vi "Remove All Trailing Zeros.vi"(1 "String in":string) -> (0 "String out":string)   [LabVIEW 2020, in "eec EST 300.lvlib"]
doc: "This utility vi takes a list of ASCII floating point numbers and removes the trailing zeros from each number."
uses:
  <instrlib>/eec EST 300/eec EST 300.lvlib
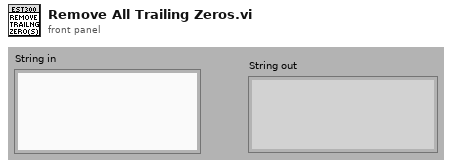
[diagram p1: front panel]
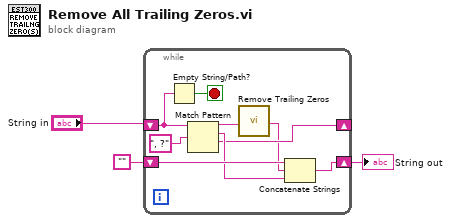
[diagram p0: block diagram]
diagram:
  n1 = while {
    shift-left: "" -> [w10]
    shift-right: [w11] -> w1
    shift-left: "String in" -> [w6]
    shift-right: [w8] -> _
    stop <- w7 stop-if-true
    n2 = Empty String/Path?(string/path=w6) -> (empty?=w7:bool)
    n3 = Match Pattern(string=w6, regular expression=", ?") -> (before substring=w5:string, match substring=w9:string, after substring=w8:string)  [unwired: 1 in, 1 out]
    n4 = call <instrlib>:"Remove Trailing Zeros.vi"("Floating Point Number"=w5) -> ("Remove Trailing Zeros"=w4:string)
    n5 = Concatenate Strings(w10, w4, w9) -> (w11:string)
  }
  "String out" <- w1
